vi "Send lfieldpanel_acquire_single_frame.vi"(5 "notes":string, 6 "savepath":path, 7 "Message Priority (Normal)":T1=enum."Normal", 8 "error in (no error)":errorcluster, 9 "Log data":bool, 10 "Integrate_sensor":bool, 11 "Message Enqueuer":refnum<class "Message Enqueuer.lvclass">) -> (0 "error out":errorcluster, 3 "Message Enqueuer out":refnum<class "Message Enqueuer.lvclass">)   [LabVIEW 2015, in "lfieldpanel_acquire_single_frame Msg.lvclass"]
doc: "This VI sends the message to an actor."
uses:
  lfieldpanel_acquire_single_frame Msg.lvclass
  <vilib>/ActorFramework/Message Enqueuer/Message Enqueuer.lvclass
  <vilib>/ActorFramework/Message Enqueuer/Message Priority.ctl
  lfieldpanel_acquire_single_frame Msg.lvclass/lfieldpanel_acquire_single_frame Msg.ctl
  <vilib>/ActorFramework/Message Enqueuer/Message Enqueuer.lvclass/Message Enqueuer.ctl
  <vilib>/ActorFramework/Message Priority Queue/Priority Enqueue.vi
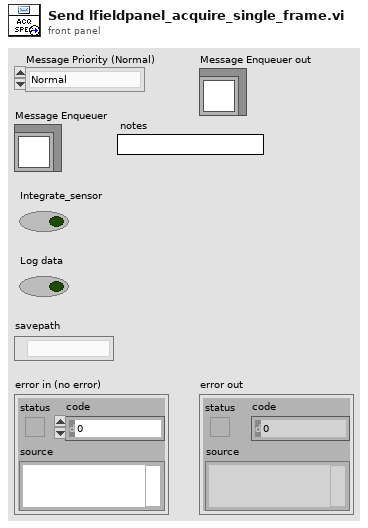
[diagram p1: front panel]
types:
  T1 = typedef "Actor Framework.lvlib/Message Enqueuer.lvclass/Message Priority.ctl" = enum16{"Low", "Normal", "High"}
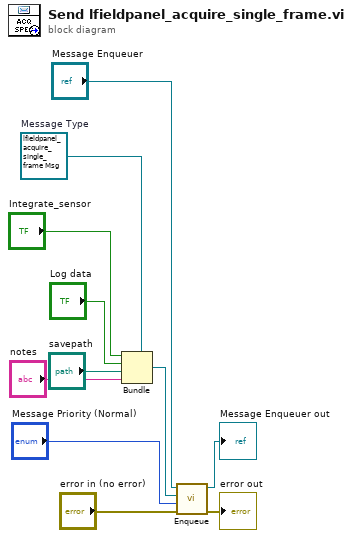
[diagram p0: block diagram]
diagram:
  w8 = refnum<class "lfieldpanel_acquire_single_frame Msg.lvclass"> refnum  # Message Type
  n1 = Bundle(cluster=w8, "Integrate_sensor", "Log data", "savepath", "notes") -> (w7:refnum<class "lfieldpanel_acquire_single_frame Msg.lvclass">)
  n2 = call <vilib>:"Enqueue.vi"("error in (no error)"="error in (no error)", "Message Priority (Normal)"="Message Priority (Normal)", "Message"=w7, "Message Enqueuer in"="Message Enqueuer") -> ("error out"=→"error out":errorcluster, "Message Enqueuer out"=→"Message Enqueuer out":refnum<class "Message Enqueuer.lvclass">)  [unwired: 6 in]
